vi "Create.vi"(8 "error in (no error)":errorcluster, 11 "pointer":i64) -> (0 "error out":errorcluster, 3 "Subscription out":refnum<class "Subscription.lvclass">)   [LabVIEW 2020, in "Client.lvlib" / "Subscription.lvclass"]
uses:
  Subscription.lvclass
  Subscription.lvclass/Subscription.ctl
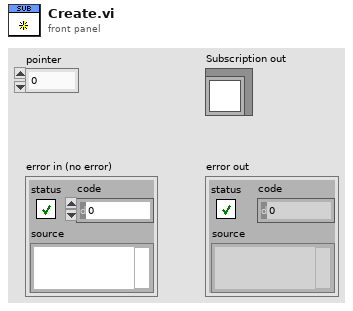
[diagram p1: front panel]
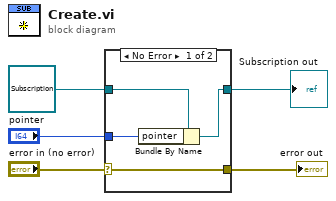
[diagram p0: block diagram]
diagram:
  n1 = case shown="No Error" "error in (no error)" {
    selector: "error in (no error)" -> [w6 w11]
    tunnel: [w6 w11] -> w4
    tunnel: [w8 w10] -> w2
    tunnel: refnum<class "Subscription.lvclass"> refnum ("Subscription in") -> [w9 w10]
    tunnel: "pointer" -> [w7 _]
    frame No Error {
      n2 = Bundle By Name(cluster=w9, "pointer"=w7) -> (w8:refnum<class "Subscription.lvclass">)
    }
    frame Error {
    }
  }
  "error out" <- w4
  "Subscription out" <- w2
